vi "data_entry_string.vi"(7 "callee":refnum<vi>, 8 "error in (no error)":errorcluster, 10 "configuration":T2, 11 "v1 in":refnum<class "v1.lvclass">) -> (0 "error out":errorcluster, 1 "data":string, 2 "dialog_selection":T1, 3 "v1 out":refnum<class "v1.lvclass">)   [LabVIEW 2015, in "lv-dialog.lvlib" / "v1.lvlib" / "v1.lvclass"]
uses:
  v1.lvclass
  _controls/dialog_selection.ctl
  _controls/error.ctl
  lv-dialog.lvlib
  v1.lvlib
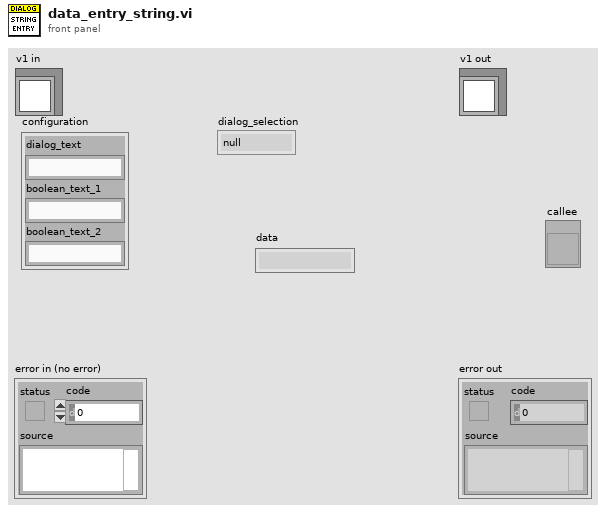
[diagram p1: front panel]
types:
  T1 = typedef "lv-dialog.lvlib/v1.lvlib/dialog_selection.ctl" = enum16{"null", "panel_closed", "button_1", "button_2", "button_3", "cancelled"}
  T2 = cluster{"dialog_text":string, "boolean_text_1":string, "boolean_text_2":string}
  T3 = typedef "lv-dialog.lvlib/error.ctl" = enum16{"null", "not_implemented"}
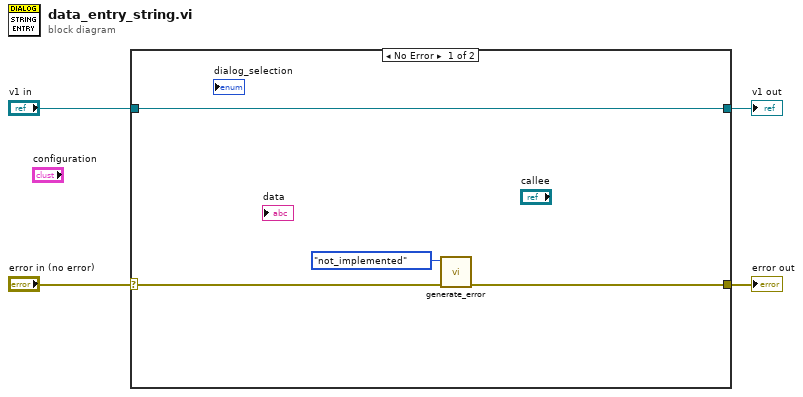
[diagram p0: block diagram]
diagram:
  n1 = case shown="No Error" "error in (no error)" {
    selector: "error in (no error)" -> [w6 w10]
    tunnel: [w5 w10] -> w3
    tunnel: [w8 w9] -> w1
    tunnel: "v1 in" -> [w8 w9]
    frame No Error {
      n2 = call "generate_error.vi"("error in (no error)"=w6, "error"=error."not_implemented") -> ("error out"=w5:errorcluster)  [unwired: 9 in]
    }
    frame Error {
    }
  }
  "error out" <- w3
  "v1 out" <- w1
